vi "Calculate merit factor.vi"(8 "error in (no error)":errorcluster, 11 "DAQOrcaFlash in":refnum<class "DAQOrcaFlash.lvclass">) -> (0 "error out":errorcluster, 3 "DAQOrcaFlash out":refnum<class "DAQOrcaFlash.lvclass">)   [LabVIEW 2012, in "DAQOrcaFlash.lvclass"]
uses:
  DAQOrcaFlash.lvclass
  ROI options.ctl
  <vilib>/Distrio/Murmex/GenericMessage/GenericMessage.lvclass
  DAQOrcaFlash.lvclass/DAQOrcaFlash.ctl
  <vilib>/Analysis/6fits.llb/Curve Fitting Criteria.ctl
  <vilib>/Analysis/baseanly.llb/Mean (DBL).vi
  <vilib>/Analysis/NI_AALBase.lvlib
  <vilib>/vision/NI_Vision_Development_Module.lvlib
  <vilib>/Analysis/NI_AALPro.lvlib
  <vilib>/Distrio/Murmex/Message/Message.lvclass
  <vilib>/Distrio/Murmex/Murmex/Murmex.lvclass
panel:
  in  "amplitude guess":dbl=1.0
  in  "STD guess":dbl=0.1
  out "LP":T1(plugin-control)
  out "HP":dbl(graph)
  out "LP":dbl(graph)
  out "y2 2":dbl
  out "x2 2":dbl
  out "y1 2":dbl
  out "x1 2":dbl
  out "parameter guesses":dbl[](array[numeric])
  out "mean":dbl format="%0.2f"
  out "min value":dbl
  out "best fit parameters":dbl[](array[numeric])
  out "XY Graph":cluster{cdb[]}[](graph)
  out "size y":i32
  out "y2":dbl
  out "x2":dbl
  out "y1":dbl
  out "x1":dbl
  out "Runtime cluster.ROI Descriptor.Global Rectangle":i32[](array[numeric])
  out "offset":dbl
  out "standard deviation":dbl
  in  "ROI options 2":T2
  out "amplitude":dbl
  out "residue":dbl
  out "center":dbl
  out "Raw data":cluster{"Y":dbl[], "Y":dbl[]}[](graph)
  out "Gauss":cluster{"Y":dbl[], "Y":dbl[]}[](graph)
  out "HP":T1(plugin-control)
  out "MF":dbl(graph)
  # "y_min"
  # "y mean"
  # "ampl"
  # "STD"
  # "xo"
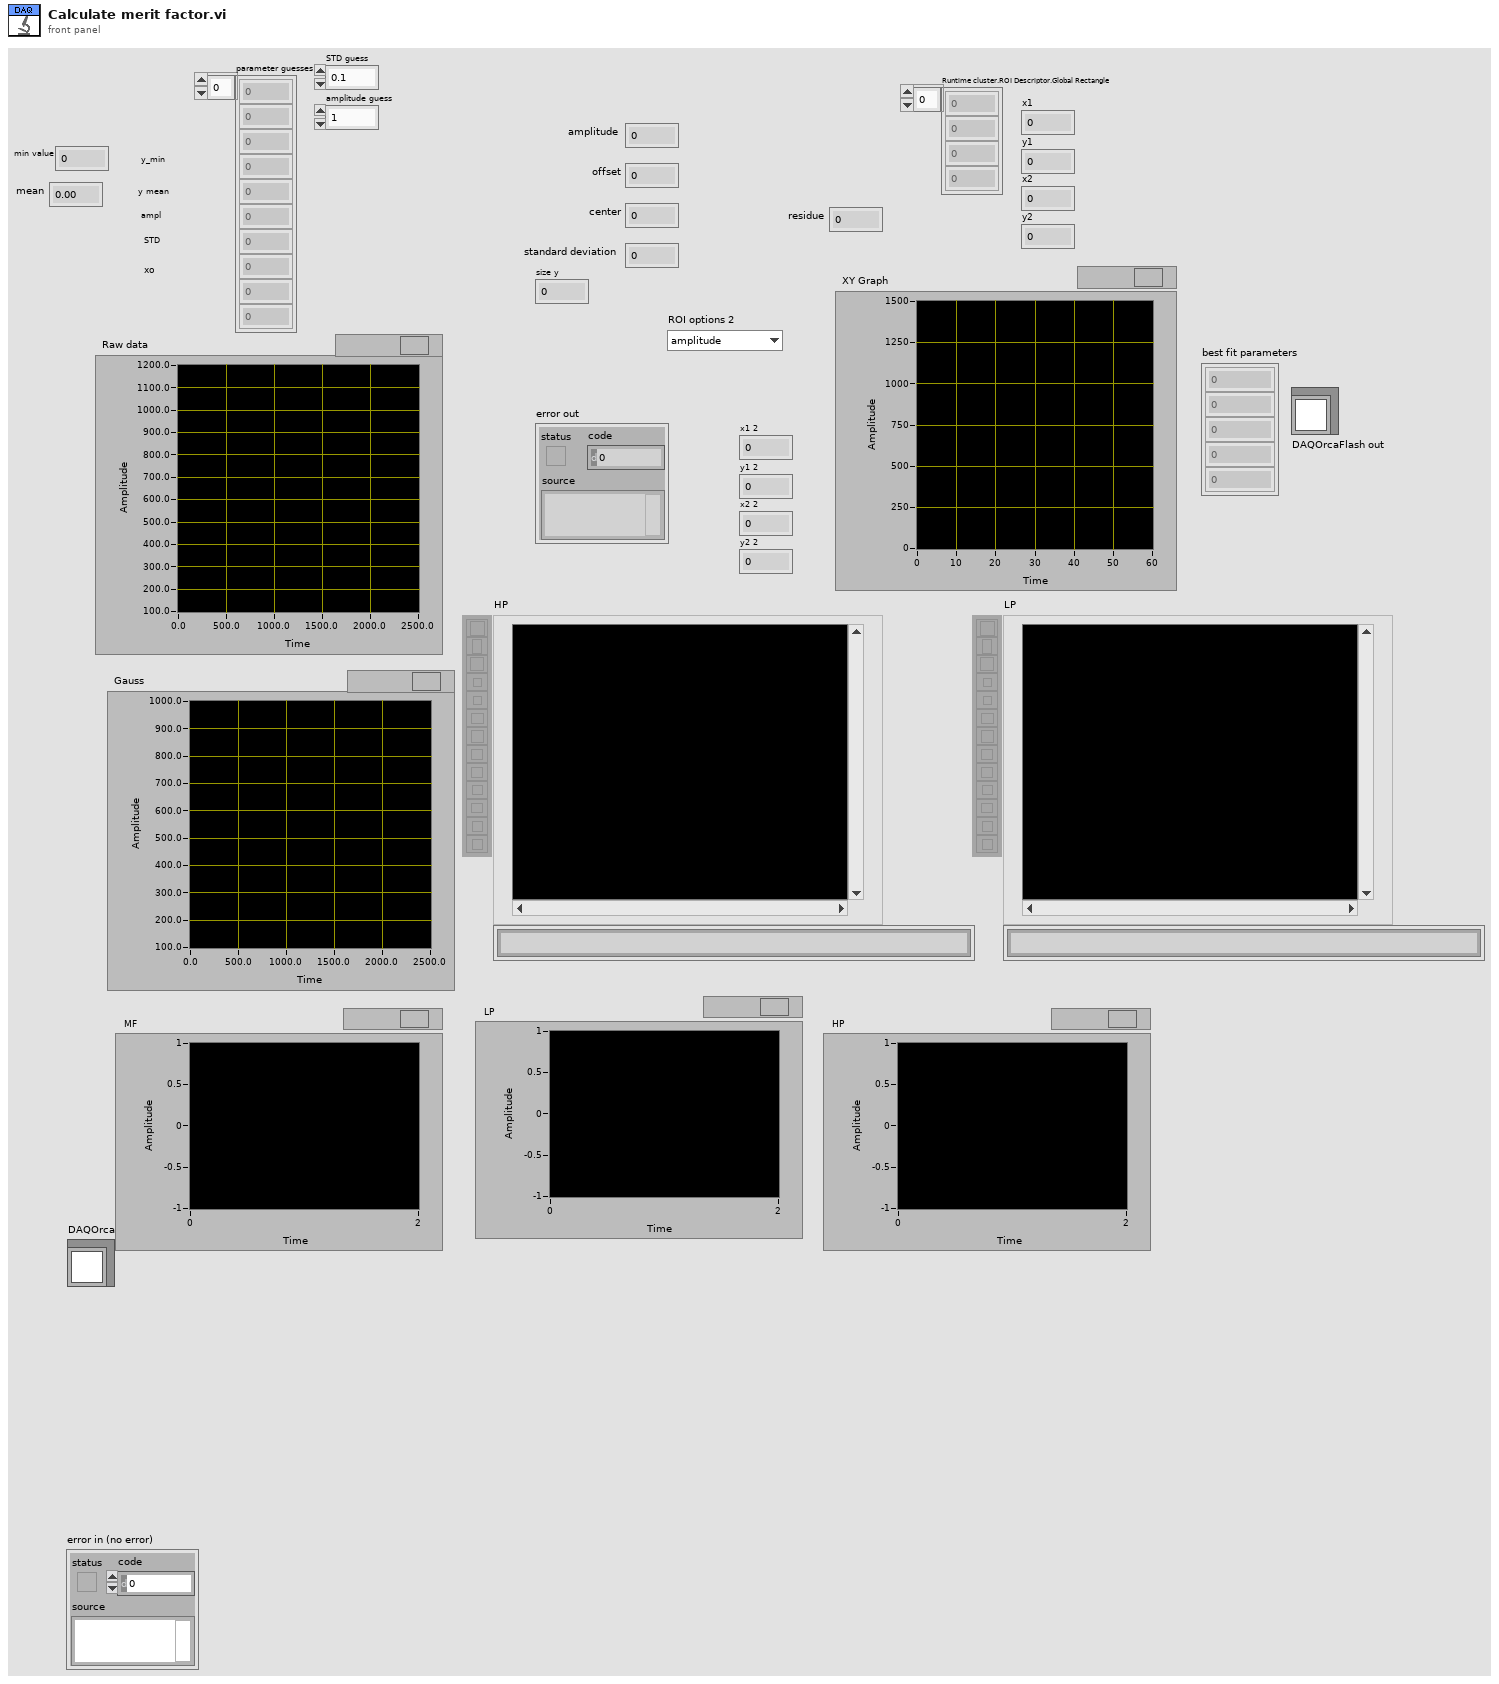
[diagram p1: front panel]
types:
  T1 = typedef "IMAQ Image.ctl" = refnum<image>
  T2 = typedef "DAQOrcaFlash.lvclass/ROI options.ctl" = enum16{"amplitude", "ERF", "residue", "amplitude/STD", "amplitude/offset"}
  T3 = cluster{"initial amplitude":dbl, "initial center":dbl, "initial standard deviation":dbl, "offset":dbl}
  T4 = cluster{"amp min":dbl, "amp max":dbl, "center min":dbl, "center max":dbl, "deviation min":dbl, "deviation max":dbl, "offset min":dbl, "offset max":dbl}
  T5 = typedef "Image Type" = u32
  T6 = typedef "DAQOrcaFlash.lvclass/merit_factor_type.ctl" = enum16{"full frame intensity", "ROI beads", "Weber contrast", "Michelson contrast", "RMS contrast", "Line profile analysis", "ROI analysis", "FFT", "SNR", "5% brightest"}
  T7 = typedef "ROI Descriptor" = cluster{"Global Rectangle":i32[], "Contours":cluster{"ID":enum32{"External", "Internal"}, "Type":u32, "Coordinates":i32[]}[]}
  T8 = cluster{"histogram":u32[], "Minimal Value":sgl, "Maximal Value":sgl, "Starting Value":sgl, "Interval Width":sgl, "Mean Value":sgl, "Standard  Variation":sgl, "Area (pixels)":i32}
  T9 = typedef "NI_AALPro.lvlib/Curve Fitting Criteria.ctl" = u16
  T10 = cluster{"Min":sgl, "Max":sgl, "Mean":sgl, "Std Dev":sgl, "Count":i32}
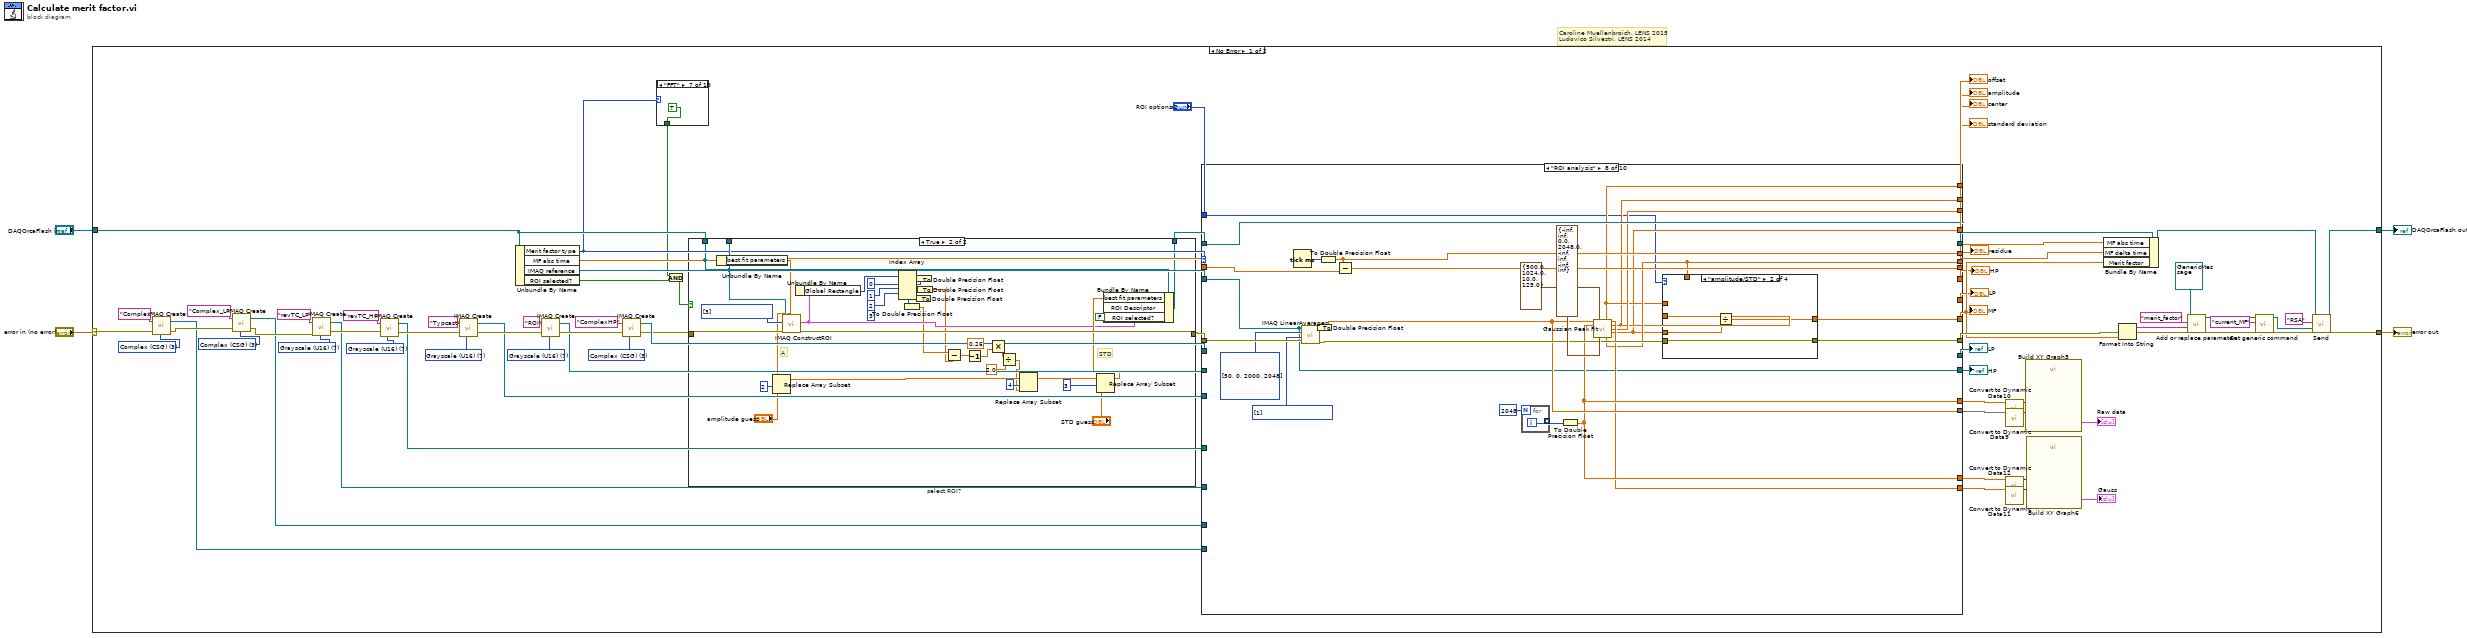
[diagram p0: block diagram]
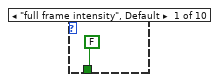
[diagram p2: hidden frame]
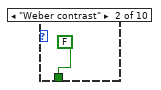
[diagram p3: hidden frame]
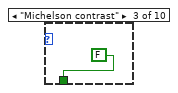
[diagram p4: hidden frame]
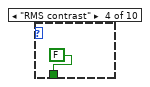
[diagram p5: hidden frame]
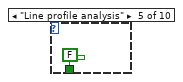
[diagram p6: hidden frame]
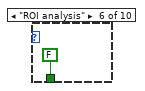
[diagram p7: hidden frame]
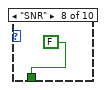
[diagram p8: hidden frame]
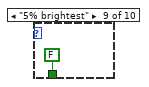
[diagram p9: hidden frame]
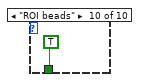
[diagram p10: hidden frame]
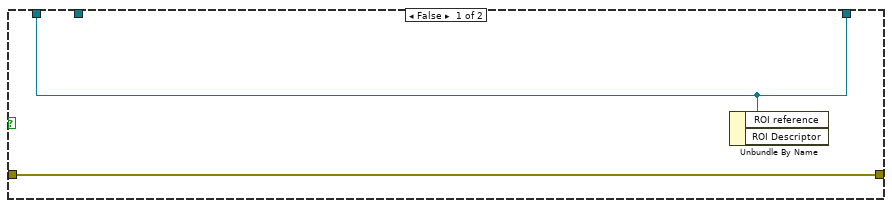
[diagram p11: hidden frame]
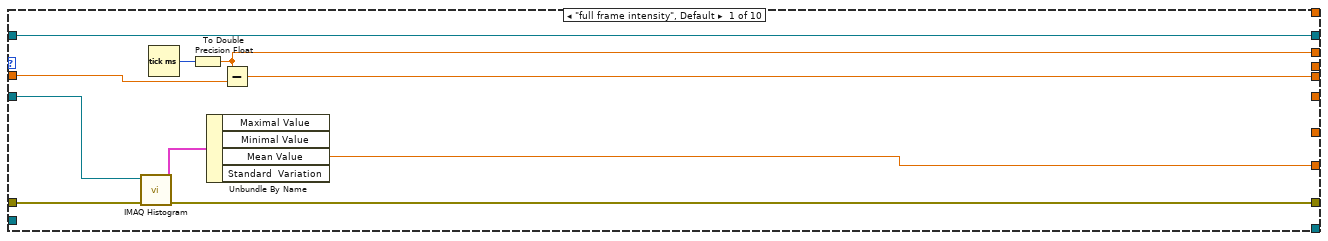
[diagram p12: hidden frame]
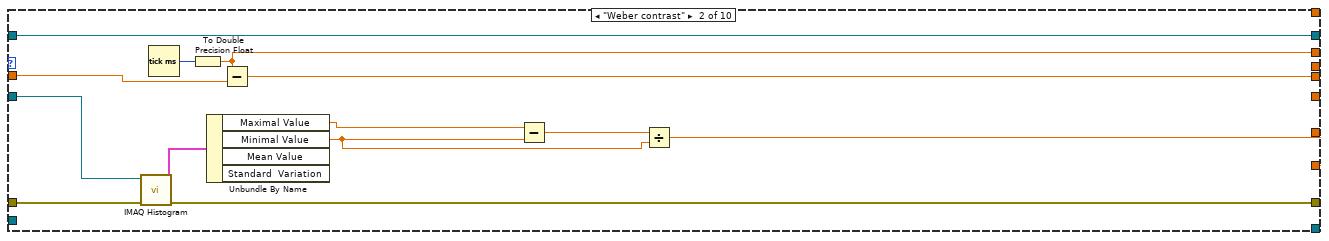
[diagram p13: hidden frame]
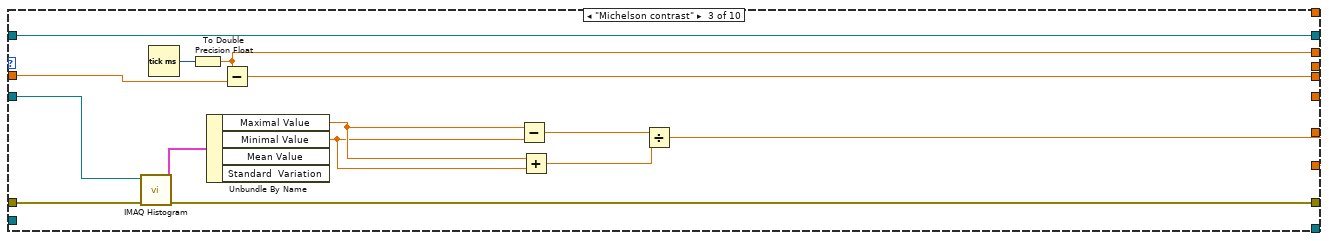
[diagram p14: hidden frame]
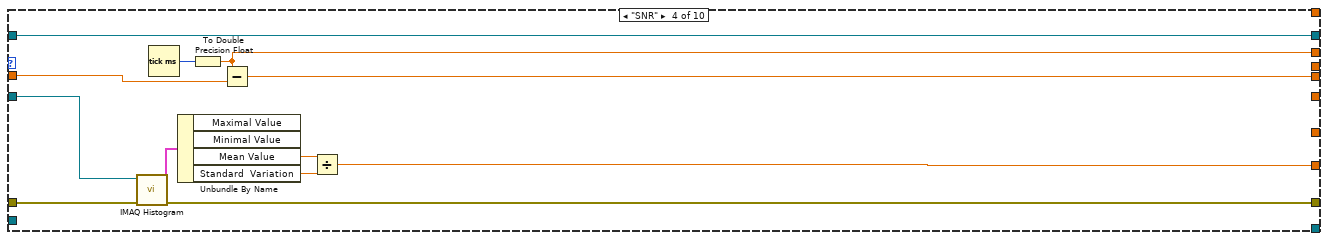
[diagram p15: hidden frame]
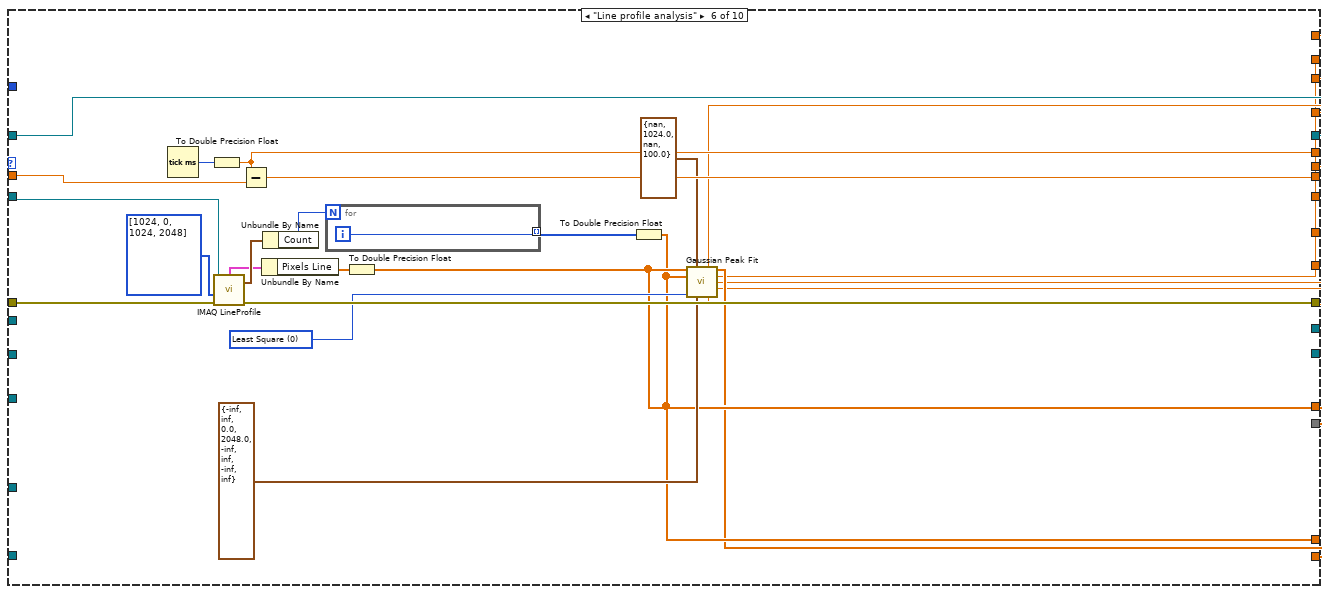
[diagram p17: hidden frame]
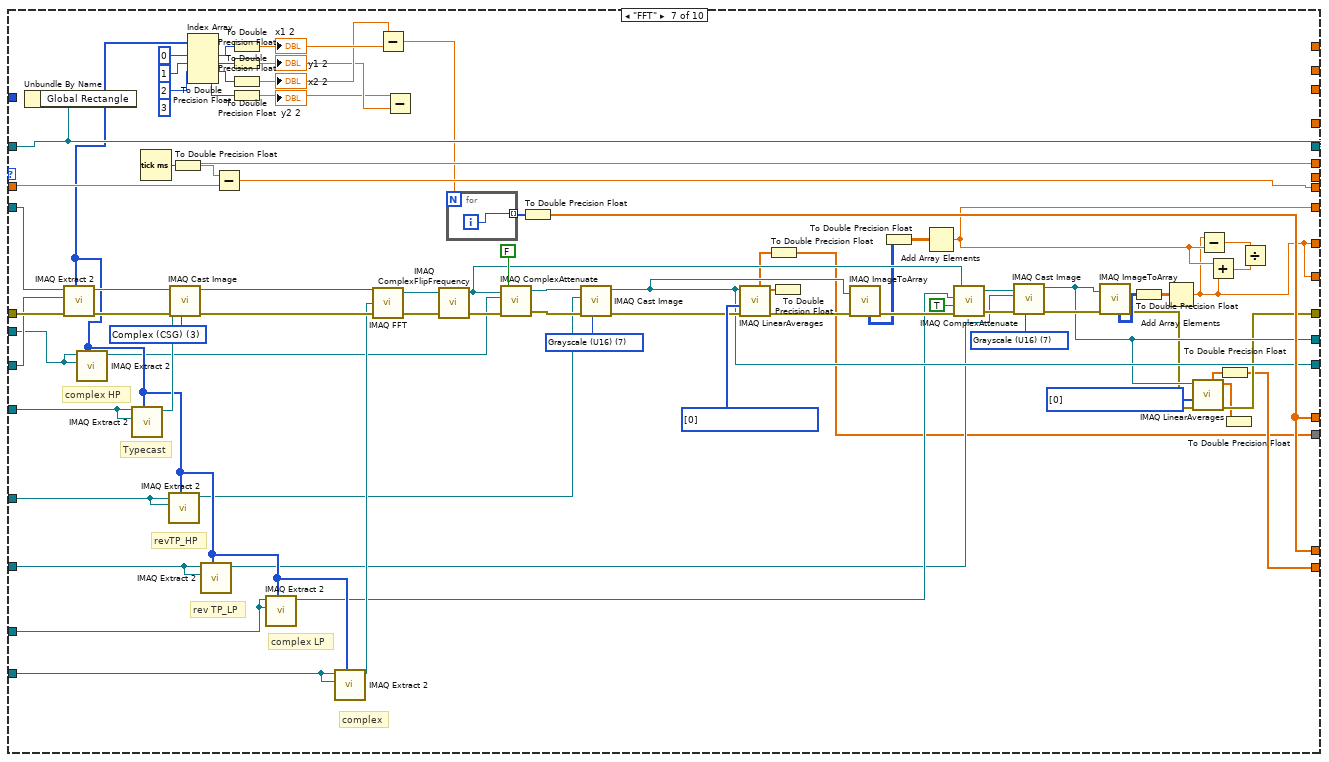
[diagram p18: hidden frame]
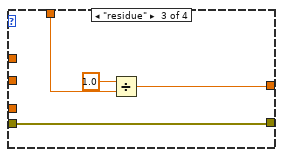
[diagram p20: hidden frame]
diagram:
  # "Caroline Muellenbroich, LENS 2015\nLudovico Silvestri, LENS 2014"
  n1 = case shown="No Error" "error in (no error)" {
    selector: "error in (no error)" -> [w11 w438]
    tunnel: [w67 w438] -> w4
    tunnel: "DAQOrcaFlash in" -> [w38 w439]
    tunnel: [w63 w439] -> w2
    frame No Error {
      w9 = T5 3 items=["Grayscale (U8)", "Grayscale (I16)", "Grayscale (SGL)", "Complex (CSG)", "RGB (U32)", "HSL (U32)", "RGB (U64)", "Grayscale (U16)"] ("Image Type")
      w14 = T5 3 items=["Grayscale (U8)", "Grayscale (I16)", "Grayscale (SGL)", "Complex (CSG)", "RGB (U32)", "HSL (U32)", "RGB (U64)", "Grayscale (U16)"] ("Image Type")
      w18 = T5 7 items=["Grayscale (U8)", "Grayscale (I16)", "Grayscale (SGL)", "Complex (CSG)", "RGB (U32)", "HSL (U32)", "RGB (U64)", "Grayscale (U16)"] ("Image Type")
      w22 = T5 7 items=["Grayscale (U8)", "Grayscale (I16)", "Grayscale (SGL)", "Complex (CSG)", "RGB (U32)", "HSL (U32)", "RGB (U64)", "Grayscale (U16)"] ("Image Type")
      w28 = T5 7 items=["Grayscale (U8)", "Grayscale (I16)", "Grayscale (SGL)", "Complex (CSG)", "RGB (U32)", "HSL (U32)", "RGB (U64)", "Grayscale (U16)"] ("Image Type")
      w31 = T5 7 items=["Grayscale (U8)", "Grayscale (I16)", "Grayscale (SGL)", "Complex (CSG)", "RGB (U32)", "HSL (U32)", "RGB (U64)", "Grayscale (U16)"] ("Image Type")
      w61 = T5 3 items=["Grayscale (U8)", "Grayscale (I16)", "Grayscale (SGL)", "Complex (CSG)", "RGB (U32)", "HSL (U32)", "RGB (U64)", "Grayscale (U16)"] ("Image Type")
      n2 = call "IMAQ Create"("Image Name"="Complex", "Image Type"=w9, "error in (no error)"=w11) -> ("New Image"=w8:T1, "error out"=w10:errorcluster)  [unwired: 2 in]
      n3 = call "IMAQ Create"("Image Name"="Complex_LP", "Image Type"=w14, "error in (no error)"=w10) -> ("New Image"=w13:T1, "error out"=w15:errorcluster)  [unwired: 2 in]
      n4 = call "IMAQ Create"("Image Name"="revTC_LP", "Image Type"=w18, "error in (no error)"=w15) -> ("New Image"=w17:T1, "error out"=w19:errorcluster)  [unwired: 2 in]
      n5 = call "IMAQ Create"("Image Name"="revTC_HP", "Image Type"=w22, "error in (no error)"=w19) -> ("New Image"=w21:T1, "error out"=w23:errorcluster)  [unwired: 2 in]
      n6 = call "IMAQ Create"("Image Name"="Typcast", "Image Type"=w28, "error in (no error)"=w23) -> ("New Image"=w25:T1, "error out"=w26:errorcluster)  [unwired: 2 in]
      n7 = Unbundle By Name(w38) -> ("Merit factor type"=w36:T6, "MF abs time"=w80:dbl, "IMAQ reference"=w55:T1, "ROI selected?"=w35:bool)
      n8 = call "IMAQ Create"("Image Name"="ROI", "Image Type"=w31, "error in (no error)"=w26) -> ("New Image"=w29:T1, "error out"=w30:errorcluster)  [unwired: 2 in]
      n9 = call "IMAQ Create"("Image Name"="ComplexHP", "Image Type"=w61, "error in (no error)"=w30) -> ("New Image"=w60:T1, "error out"=w57:errorcluster)  [unwired: 2 in]
      n10 = case shown="\"FFT\"" w36 {
        tunnel: [FALSE FALSE FALSE FALSE FALSE FALSE TRUE FALSE FALSE TRUE] -> w34
        frame "full frame intensity", Default {
        }
        frame "Weber contrast" {
        }
        frame "Michelson contrast" {
        }
        frame "RMS contrast" {
        }
        frame "Line profile analysis" {
        }
        frame "ROI analysis" {
        }
        frame "FFT" {
        }
        frame "SNR" {
        }
        frame "5% brightest" {
        }
        frame "ROI beads" {
        }
      }
      n11 = And(x=w34, y=w35) -> (x .and. y?=w33:bool)
      n12 = case "select ROI?" shown="True" w33 {
        tunnel: w57 -> [w92 w124]
        tunnel: [w92 w123] -> w56
        tunnel: w55 -> [_ w122]
        tunnel: w38 -> [w91 w119]
        tunnel: [w91 w121] -> w37
        frame False {
          n13 = Unbundle By Name(w91) -> ()  [unwired: 2 out]
        }
        frame True {
          (unwired) 3 ("index")
          w125 = u32[] [3] items=["No Selection", "Point", "Line", "Rectangle", "Oval", "Polygon", "Freehand Region", "Annulus", "Zoom", "Pan", "Broken Line", "Freehand Line", "Rotated Rectangle"] ("Tools")
          # "A"
          # "STD"
          n14 = Unbundle By Name(w119) -> ("best fit parameters"=w114:dbl[])
          n15 = Replace Array Subset(array=w114, new element="amplitude guess", index=2) -> (w99:dbl[])
          n16 = call "IMAQ ConstructROI"("error in (no error)"=w124, "Tools"=w125, "Image"=w122) -> ("error out"=w123:errorcluster, "ROI Descriptor Out"=w112:T7)  [unwired: 5 in, 2 out]
          n17 = Unbundle By Name(w112) -> ("Global Rectangle"=w104:i32[])
          n18 = Index Array(array=w104, index #1=0 ("index"), index #2=1 ("index"), index #3=2 ("index")) -> (element #1=w111:i32, element #2=w110:i32, element #3=w108:i32, element #4=w109:i32)  [unwired: 1 in]
          n19 = To Double Precision Float(number=w109) -> (double precision float=w103:dbl)
          n20 = To Double Precision Float(number=w108) -> ()  [unwired: 1 out]
          n21 = To Double Precision Float(number=w111) -> ()  [unwired: 1 out]
          n22 = To Double Precision Float(number=w110) -> (double precision float=w102:dbl)
          n23 = Subtract(x=w103, y=w102) -> (x-y=w101:dbl)
          n24 = Decrement(x=w101) -> (x-1=w94:dbl)
          n25 = Multiply(x=0.26, y=w94) -> (x*y=w93:dbl)
          n26 = Divide(x=w93, y=2.0) -> (x/y=w96:dbl)
          n27 = Replace Array Subset(array=w99, new element=w96, index=4) -> (w98:dbl[])
          n28 = Replace Array Subset(array=w98, new element="STD guess", index=3) -> (w113:dbl[])
          n29 = Bundle By Name(cluster=w119, "best fit parameters"=w113, "ROI Descriptor"=w112, "ROI selected?"=FALSE ("Runtime cluster.ROI selected?")) -> (w121:refnum<class "DAQOrcaFlash.lvclass">)
        }
      }
      n30 = case shown="\"ROI analysis\"" w36 {
        tunnel: [w129 w142 w156 w168 w175 w199 w229 w292 w363 w418] -> w74
        tunnel: w56 -> [w130 w143 w157 w169 w175 w201 w264 w299 w355 w417]
        tunnel: w37 -> [w132 w145 w159 w171 w176 w194 w265 w305 w325 w416]
        tunnel: [w132 w145 w159 w171 w176 w194 w265 w305 w324 w416] -> w78
        tunnel: w80 -> [w135 w148 w162 w174 _ w190 w266 w302 w370 w415]
        tunnel: [w134 w147 w161 w173 _ w189 w259 w301 w369 w414] -> w79
        tunnel: [w126 w136 w152 w163 _ w177 w203 w291 w362 w413] -> w62
        tunnel: [w131 w144 w158 w170 _ w188 w257 w300 w368 w412] -> w77
        tunnel: w55 -> [w128 w141 w155 w167 _ w200 w262 w281 w346 _]
        tunnel: w60 -> [_ _ _ _ _ _ w224 _ _ _]
        tunnel: [_ _ _ _ _ _ w239 w281 w345 _] -> w58
        tunnel: [_ _ _ _ _ w182 w253 w289 w321 _] -> w48
        tunnel: [_ _ _ _ _ w183 w206 w290 w327 _] -> w47
        tunnel: [_ _ _ _ _ w182 w253 w289 w321 _] -> w46
        tunnel: [_ _ _ _ _ w181 w207 w288 w329 _] -> w45
        tunnel: [_ _ _ _ _ w184 _ w285 w361 _] -> w44
        tunnel: [_ _ _ _ _ w177 _ w284 w360 _] -> w43
        tunnel: [_ _ _ _ _ w180 _ w286 w359 _] -> w42
        tunnel: [_ _ _ _ _ w179 _ w283 w358 _] -> w41
        tunnel: [_ _ _ _ _ w178 _ w287 w357 _] -> w40
        tunnel: "ROI options 2" -> [_ _ _ _ _ _ _ w282 w356 _]
        tunnel: w29 -> [_ _ _ _ _ _ w263 _ w343 _]
        tunnel: w25 -> [_ _ _ _ _ _ w223 _ _ _]
        tunnel: w21 -> [_ _ _ _ _ _ w221 _ _ _]
        tunnel: w17 -> [_ _ _ _ _ _ w220 _ _ _]
        tunnel: w13 -> [_ _ _ _ _ _ w219 _ _ _]
        tunnel: w8 -> [_ _ _ _ _ _ w218 _ _ _]
        tunnel: [_ _ _ _ _ _ w231 _ _ _] -> w7
        tunnel: [_ _ _ _ _ _ w204 _ _ _] -> w6
        tunnel: [_ _ _ _ _ _ w203 _ _ _] -> w5
        frame "full frame intensity", Default {
          n31 = call "IMAQ Histogram"("error in (no error)"=w130, "Image"=w128) -> ("error out"=w129:errorcluster, "Histogram Report"=w127:T8)  [unwired: 8 in]
          n32 = Tick Count (ms)() -> (millisecond timer value=w133:u32)
          n33 = To Double Precision Float(number=w133) -> (double precision float=w131:dbl)
          n34 = Unbundle By Name(w127) -> ("Mean Value"=w126:sgl)  [unwired: 3 out]
          n35 = Subtract(x=w131, y=w135) -> (x-y=w134:dbl)
        }
        frame "Weber contrast" {
          n36 = call "IMAQ Histogram"("error in (no error)"=w143, "Image"=w141) -> ("error out"=w142:errorcluster, "Histogram Report"=w140:T8)  [unwired: 8 in]
          n37 = Tick Count (ms)() -> (millisecond timer value=w146:u32)
          n38 = To Double Precision Float(number=w146) -> (double precision float=w144:dbl)
          n39 = Unbundle By Name(w140) -> ("Maximal Value"=w139:sgl, "Minimal Value"=w137:sgl)  [unwired: 2 out]
          n40 = Subtract(x=w144, y=w148) -> (x-y=w147:dbl)
          n41 = Subtract(x=w139, y=w137) -> (x-y=w138:sgl)
          n42 = Divide(x=w138, y=w137) -> (x/y=w136:sgl)
        }
        frame "Michelson contrast" {
          n43 = call "IMAQ Histogram"("error in (no error)"=w157, "Image"=w155) -> ("error out"=w156:errorcluster, "Histogram Report"=w154:T8)  [unwired: 8 in]
          n44 = Tick Count (ms)() -> (millisecond timer value=w160:u32)
          n45 = To Double Precision Float(number=w160) -> (double precision float=w158:dbl)
          n46 = Unbundle By Name(w154) -> ("Maximal Value"=w151:sgl, "Minimal Value"=w150:sgl)  [unwired: 2 out]
          n47 = Subtract(x=w158, y=w162) -> (x-y=w161:dbl)
          n48 = Subtract(x=w151, y=w150) -> (x-y=w153:sgl)
          n49 = Add(x=w151, y=w150) -> (x+y=w149:sgl)
          n50 = Divide(x=w153, y=w149) -> (x/y=w152:sgl)
        }
        frame "SNR" {
          n51 = call "IMAQ Histogram"("error in (no error)"=w169, "Image"=w167) -> ("error out"=w168:errorcluster, "Histogram Report"=w166:T8)  [unwired: 8 in]
          n52 = Tick Count (ms)() -> (millisecond timer value=w172:u32)
          n53 = Unbundle By Name(w166) -> ("Mean Value"=w165:sgl, "Standard  Variation"=w164:sgl)  [unwired: 2 out]
          n54 = To Double Precision Float(number=w172) -> (double precision float=w170:dbl)
          n55 = Subtract(x=w170, y=w174) -> (x-y=w173:dbl)
          n56 = Divide(x=w165, y=w164) -> (x/y=w163:sgl)
        }
        frame "RMS contrast" {
        }
        frame "Line profile analysis" {
          w187 = T9 0 items=["Least Square", "Least Absolute Residual", "Bisquare"] ("method")
          n57 = Tick Count (ms)() -> (millisecond timer value=w191:u32)
          n58 = To Double Precision Float(number=w191) -> (double precision float=w188:dbl)
          n59 = call "IMAQ LineProfile"("error in (no error)"=w201, "Line Coordinates"=i32[] [1024, 0, 1024, 2048], "Image"=w200) -> ("error out"=w199:errorcluster, "Line Graph"=w196:cluster{"x0":sgl, "dx":sgl, "Pixels Line":sgl[]}, "Line Information"=w198:T10)  [unwired: 2 in, 1 out]
          n60 = Subtract(x=w188, y=w190) -> (x-y=w189:dbl)
          n61 = Unbundle By Name(w196) -> ("Pixels Line"=w195:sgl[])
          n62 = Unbundle By Name(w198) -> ("Count"=w193:i32)
          n63 = for {
            N: w193 -> [_]
            tunnel: [w202] -> w192 mode=indexing
            i -> [w202]
          }
          n64 = To Double Precision Float(number=w195) -> (double precision float=w183:dbl[])
          n65 = To Double Precision Float(number=w192) -> (double precision float=w182:dbl[])
          n66 = call <vilib>:"Gaussian Peak Fit.vi"("Y"=w183, "initial guess"=T3 {"initial amplitude"=nan, "initial center"=1024.0, "initial standard deviation"=nan, "offset"=100.0}, "X"=w182, "method"=w187, "parameter bounds"=T4 {"amp min"=-inf, "amp max"=inf, "center min"=0.0, "center max"=2048.0, "deviation min"=-inf, "deviation max"=inf, "offset min"=-inf, "offset max"=inf}) -> ("offset"=w184:dbl, "Best Gaussian Fit"=w181:dbl[], "amplitude"=w177:dbl, "center"=w180:dbl, "standard deviation"=w179:dbl, "residue"=w178:dbl)  [unwired: 4 in, 1 out]
        }
        frame "FFT" {
          w228 = i32[] [0] items=["X Axis Averages", "Y Axis Averages", "X + Y Axis Averages", "X - Y Axis Averages"] ("Averages")
          w243 = T5 7 items=["Grayscale (U8)", "Grayscale (I16)", "Grayscale (SGL)", "Complex (CSG)", "RGB (U32)", "HSL (U32)", "RGB (U64)", "Grayscale (U16)"] ("Image Type")
          w254 = T5 7 items=["Grayscale (U8)", "Grayscale (I16)", "Grayscale (SGL)", "Complex (CSG)", "RGB (U32)", "HSL (U32)", "RGB (U64)", "Grayscale (U16)"] ("Image Type")
          w261 = i32[] [0] items=["X Axis Averages", "Y Axis Averages", "X + Y Axis Averages", "X - Y Axis Averages"] ("Averages")
          (unwired) 3 ("index")
          w278 = T5 3 items=["Grayscale (U8)", "Grayscale (I16)", "Grayscale (SGL)", "Complex (CSG)", "RGB (U32)", "HSL (U32)", "RGB (U64)", "Grayscale (U16)"] ("Image Type")
          # "complex"
          # "complex LP"
          # "rev TP_LP"
          # "revTP_HP"
          # "Typecast"
          # "complex HP"
          n67 = Unbundle By Name(w265) -> ("Global Rectangle"=w217:i32[])
          n68 = call "IMAQ Extract 2"("Optional Rectangle"=w217, "error in (no error)"=w264, "Image Dst"=w263, "Image Src"=w262) -> ("error out"=w226:errorcluster, "Image Dst Out"=w227:T1)  [unwired: 6 in]
          n69 = call "IMAQ Extract 2"("Optional Rectangle"=w217, "Image Dst"=w224, "Image Src"=w224) -> ("Image Dst Out"=w214:T1)  [unwired: 7 in, 1 out]
          n70 = call "IMAQ Extract 2"("Optional Rectangle"=w217, "Image Dst"=w223, "Image Src"=w223) -> ("Image Dst Out"=w222:T1)  [unwired: 7 in, 1 out]
          n71 = Tick Count (ms)() -> (millisecond timer value=w258:u32)
          n72 = call "IMAQ Extract 2"("Optional Rectangle"=w217, "Image Dst"=w221, "Image Src"=w221) -> ("Image Dst Out"=w213:T1)  [unwired: 7 in, 1 out]
          n73 = call "IMAQ Cast Image"("Image Type"=w278, "error in (no error)"=w226, "Image Dst"=w222, "Image Src"=w227) -> ("error out"=w225:errorcluster, "Image Dst Out"=w216:T1)  [unwired: 6 in]
          n74 = To Double Precision Float(number=w258) -> (double precision float=w257:dbl)
          n75 = Index Array(array=w217, index #1=0 ("index"), index #2=1 ("index"), index #3=2 ("index")) -> (element #1=w270:i32, element #2=w271:i32, element #3=w273:i32, element #4=w272:i32)  [unwired: 1 in]
          n76 = call "IMAQ Extract 2"("Optional Rectangle"=w217, "Image Dst"=w220, "Image Src"=w220) -> ("Image Dst Out"=w211:T1)  [unwired: 7 in, 1 out]
          n77 = Subtract(x=w257, y=w266) -> (x-y=w259:dbl)
          n78 = To Double Precision Float(number=w270) -> (double precision float=w269:dbl)
          "x1 2" <- w269
          n79 = To Double Precision Float(number=w271) -> (double precision float=w267:dbl)
          "y1 2" <- w267
          n80 = To Double Precision Float(number=w273) -> (double precision float=w268:dbl)
          "x2 2" <- w268
          n81 = To Double Precision Float(number=w272) -> (double precision float=w256:dbl)
          "y2 2" <- w256
          n82 = call "IMAQ Extract 2"("Optional Rectangle"=w217, "Image Dst"=w219, "Image Src"=w219) -> ("Image Dst Out"=w212:T1)  [unwired: 7 in, 1 out]
          n83 = call "IMAQ Extract 2"("Optional Rectangle"=w217, "Image Dst"=w218, "Image Src"=w218) -> ("Image Dst Out"=w215:T1)  [unwired: 7 in, 1 out]
          n84 = call "IMAQ FFT"("error in (no error)"=w225, "Image Dst"=w215, "Image Src"=w216) -> ("error out"=w252:errorcluster, "Image Dst Out"=w251:T1)  [unwired: 1 in]
          n85 = Subtract(x=w268, y=w269) -> (x-y=w205:dbl)
          n86 = Subtract(x=w256, y=w267) -> ()  [unwired: 1 out]
          n87 = call "IMAQ ComplexFlipFrequency"("error in (no error)"=w252, "Image Src"=w251) -> ("error out"=w250:errorcluster, "Image Dst Out"=w246:T1)  [unwired: 2 in]
          n88 = for {
            N: w205 -> [_]
            tunnel: [w279] -> w277 mode=indexing
            i -> [w279]
          }
          n89 = call "IMAQ ComplexAttenuate"("error in (no error)"=w250, "Low pass/High pass (Low pass)"=FALSE, "Image Dst"=w214, "Image Src"=w246) -> ("error out"=w249:errorcluster, "Image Dst Out"=w248:T1)  [unwired: 1 in]
          n90 = To Double Precision Float(number=w277) -> (double precision float=w253:dbl[])
          n91 = call "IMAQ Cast Image"("Image Type"=w254, "error in (no error)"=w249, "Image Dst"=w213, "Image Src"=w248) -> ("error out"=w255:errorcluster, "Image Dst Out"=w239:T1)  [unwired: 6 in]
          n92 = call "IMAQ LinearAverages"("error in (no error)"=w255, "Averages"=w261, "Image Src"=w239) -> ("error out"=w241:errorcluster, "Y Axis Averages"=w260:sgl[], "X Axis Averages"=w210:sgl[])  [unwired: 4 in, 2 out]
          n93 = To Double Precision Float(number=w210) -> (double precision float=w206:dbl[])
          n94 = To Double Precision Float(number=w260) -> ()  [unwired: 1 out]
          n95 = call "IMAQ ImageToArray"("error in (no error)"=w241, "Image"=w239) -> ("Image Pixels (U16)"=w235:u16[][], "error out"=w240:errorcluster)  [unwired: 2 in, 3 out]
          n96 = To Double Precision Float(number=w235) -> (double precision float=w238:dbl[][])
          n97 = Add Array Elements(numeric array=w238) -> (sum=w204:dbl)
          n98 = call "IMAQ ComplexAttenuate"("error in (no error)"=w240, "Low pass/High pass (Low pass)"=TRUE, "Image Dst"=w212, "Image Src"=w246) -> ("error out"=w245:errorcluster, "Image Dst Out"=w244:T1)  [unwired: 1 in]
          n99 = call "IMAQ Cast Image"("Image Type"=w243, "error in (no error)"=w245, "Image Dst"=w211, "Image Src"=w244) -> ("error out"=w237:errorcluster, "Image Dst Out"=w231:T1)  [unwired: 6 in]
          n100 = call "IMAQ ImageToArray"("error in (no error)"=w237, "Image"=w231) -> ("Image Pixels (U16)"=w234:u16[][], "error out"=w230:errorcluster)  [unwired: 2 in, 3 out]
          n101 = To Double Precision Float(number=w234) -> (double precision float=w236:dbl[][])
          n102 = Add Array Elements(numeric array=w236) -> (sum=w203:dbl)
          n103 = call "IMAQ LinearAverages"("error in (no error)"=w230, "Averages"=w228, "Image Src"=w231) -> ("error out"=w229:errorcluster, "Y Axis Averages"=w209:sgl[], "X Axis Averages"=w208:sgl[])  [unwired: 4 in, 2 out]
          n104 = Subtract(x=w203, y=w204) -> (x-y=w232:dbl)
          n105 = Add(x=w204, y=w203) -> (x+y=w233:dbl)
          n106 = To Double Precision Float(number=w208) -> (double precision float=w207:dbl[])
          n107 = To Double Precision Float(number=w209) -> ()  [unwired: 1 out]
          n108 = Divide(x=w232, y=w233) -> ()  [unwired: 1 out]
        }
        frame "ROI analysis" {
          w297 = i32[] [1] items=["X Axis Averages", "Y Axis Averages", "X + Y Axis Averages", "X - Y Axis Averages"] ("Averages")
          n109 = Tick Count (ms)() -> (millisecond timer value=w303:u32)
          n110 = call "IMAQ LinearAverages"("error in (no error)"=w299, "Averages"=w297, "Optional Rectangle"=i32[] [50, 0, 2000, 2048], "Image Src"=w281) -> ("error out"=w293:errorcluster, "Y Axis Averages"=w295:sgl[])  [unwired: 3 in, 3 out]
          n111 = To Double Precision Float(number=w295) -> (double precision float=w290:dbl[])
          n112 = To Double Precision Float(number=w303) -> (double precision float=w300:dbl)
          n113 = Subtract(x=w300, y=w302) -> (x-y=w301:dbl)
          n114 = for {
            N: 2048 -> [_]
            tunnel: [w320] -> w304 mode=indexing
            i -> [w320]
          }
          n115 = To Double Precision Float(number=w304) -> (double precision float=w289:dbl[])
          n116 = call <vilib>:"Gaussian Peak Fit.vi"("Y"=w290, "initial guess"=T3 {"initial amplitude"=500.0, "initial center"=1024.0, "initial standard deviation"=10.0, "offset"=125.0}, "X"=w289, "parameter bounds"=T4 {"amp min"=-inf, "amp max"=inf, "center min"=0.0, "center max"=2048.0, "deviation min"=-inf, "deviation max"=inf, "offset min"=-inf, "offset max"=inf}) -> ("offset"=w285:dbl, "Best Gaussian Fit"=w288:dbl[], "amplitude"=w284:dbl, "center"=w286:dbl, "standard deviation"=w283:dbl, "residue"=w287:dbl)  [unwired: 5 in, 1 out]
          n117 = case shown="\"amplitude/STD\"" w282 {
            tunnel: w293 -> [w306 w311 w313 w316]
            tunnel: [w306 w311 w313 w316] -> w292
            tunnel: [w307 w308 w314 w317] -> w291
            tunnel: w284 -> [w307 w310 _ w319]
            tunnel: w283 -> [_ w309 _ _]
            tunnel: w285 -> [_ _ _ w318]
            tunnel: w287 -> [_ _ w315 _]
            frame "amplitude", Default {
            }
            frame "amplitude/STD" {
              n118 = Divide(x=w310, y=w309) -> (x/y=w308:dbl)
            }
            frame "residue" {
              n119 = Divide(x=1.0, y=w315) -> (x/y=w314:dbl)
            }
            frame "amplitude/offset" {
              n120 = Divide(x=w319, y=w318) -> (x/y=w317:dbl)
            }
          }
        }
        frame "ROI beads" {
          w367 = i32[] [1] items=["X Axis Averages", "Y Axis Averages", "X + Y Axis Averages", "X - Y Axis Averages"] ("Averages")
          n121 = Unbundle By Name(w325) -> ("best fit parameters"=w326:dbl[], "Global Rectangle"=w332:i32[])
          "Runtime cluster.ROI Descriptor.Global Rectangle" <- w332
          n122 = Tick Count (ms)() -> (millisecond timer value=w371:u32)
          n123 = To Double Precision Float(number=w371) -> (double precision float=w368:dbl)
          n124 = Index Array(array=w332, index #1=0 ("index"), index #2=1 ("index"), index #3=2 ("index"), index #4=3 ("index")) -> (element #1=w342:i32, element #2=w347:i32, element #3=w349:i32, element #4=w348:i32)
          n125 = Subtract(x=w368, y=w370) -> (x-y=w369:dbl)
          n126 = To Double Precision Float(number=w348) -> (double precision float=w340:dbl)
          "y2" <- w340
          n127 = To Double Precision Float(number=w349) -> (double precision float=w339:dbl)
          "x2" <- w339
          n128 = To Double Precision Float(number=w342) -> (double precision float=w341:dbl)
          "x1" <- w341
          n129 = To Double Precision Float(number=w347) -> (double precision float=w333:dbl)
          "y1" <- w333
          n130 = Subtract(x=w339, y=w341) -> ()  [unwired: 1 out]
          n131 = Subtract(x=w340, y=w333) -> (x-y=w328:dbl)
          n132 = call "IMAQ Extract 2"("Optional Rectangle"=w332, "error in (no error)"=w355, "Image Dst"=w343, "Image Src"=w346) -> ("error out"=w354:errorcluster, "Image Dst Out"=w345:T1)  [unwired: 6 in]
          n133 = call "IMAQ LinearAverages"("error in (no error)"=w354, "Averages"=w367, "Image Src"=w345) -> ("error out"=w364:errorcluster, "Y Axis Averages"=w366:sgl[], "X Axis Averages"=w331:sgl[])  [unwired: 4 in, 2 out]
          n134 = for {
            N: w328 -> [_]
            tunnel: [w410] -> w321 mode=indexing
            i -> [w409]
            n135 = To Double Precision Float(number=w409) -> (double precision float=w408:dbl)
            n136 = Multiply(x=0.26, y=w408) -> (x*y=w410:dbl)
          }
          n137 = To Double Precision Float(number=w331) -> ()  [unwired: 1 out]
          n138 = To Double Precision Float(number=w366) -> (double precision float=w330:dbl[])
          n139 = Reverse 1D Array(array=w330) -> (reversed array=w327:dbl[])
          n140 = Array Size(array=w327) -> (size(s)=→"size y":i32)
          n141 = Array Max & Min(array=w327) -> (min value=w337:dbl)  [unwired: 3 out]
          "min value" <- w337
          n142 = call-poly <vilib>:"Mean.vi"("X"=w327) -> ("mean"=w334:dbl)  [unwired: 1 out]
          "mean" <- w334
          n143 = call <vilib>:"Gaussian Peak Fit.vi"("Y"=w327, "X"=w321, "parameter bounds"=T4 {"amp min"=-inf, "amp max"=inf, "center min"=0.0, "center max"=inf, "deviation min"=-inf, "deviation max"=inf, "offset min"=-inf, "offset max"=inf}) -> ("offset"=w361:dbl, "Best Gaussian Fit"=w329:dbl[], "amplitude"=w360:dbl, "center"=w359:dbl, "standard deviation"=w358:dbl, "residue"=w357:dbl)  [unwired: 6 in, 1 out]
          n144 = Replace Array Subset(array=w326, new element=w337, index=0) -> (w336:dbl[])
          n145 = Replace Array Subset(array=w336, new element=w334, index=1) -> (w322:dbl[])
          "parameter guesses" <- w322
          n146 = case shown="\"ERF\"" w356 {
            tunnel: w364 -> [w372 w377 w379 w383 w404]
            tunnel: [w372 w377 w379 w388 w404] -> w363
            tunnel: [w373 w374 w380 w384 w405] -> w362
            tunnel: w360 -> [w373 w376 _ _ w407]
            tunnel: w358 -> [_ w375 _ _ _]
            tunnel: w361 -> [_ _ _ _ w406]
            tunnel: w357 -> [_ _ w381 _ _]
            tunnel: w321 -> [_ _ _ w387 _]
            tunnel: w327 -> [_ _ _ w386 _]
            tunnel: w322 -> [_ _ _ w385 _]
            tunnel: [_ _ _ w382 _] -> w323
            frame "amplitude", Default {
            }
            frame "amplitude/STD" {
              n147 = Divide(x=w376, y=w375) -> (x/y=w374:dbl)
            }
            frame "residue" {
              n148 = Divide(x=1.0, y=w381) -> (x/y=w380:dbl)
            }
            frame "ERF" {
              n149 = case shown="No Error" w383 {
                selector: w383 -> [w393 w403]
                tunnel: [w389 w403] -> w388
                tunnel: w387 -> [w398 _]
                tunnel: w386 -> [w397 _]
                tunnel: [w396 _] -> w382
                tunnel: w385 -> [w394 _]
                tunnel: [w391 _] -> w384
                frame No Error {
                  n150 = call "Linespread_Function.vi"("error in (no error)"=w393, "Paramter guess"=w394, "y"=w397, "x"=w398) -> ("error out"=w392:errorcluster, "XY Graph"=→"XY Graph":cluster{cdb[]}[], "best fit parameters"=w396:dbl[])  [unwired: 5 in]
                  n151 = Index Array(array=w396, index=3) -> (element=w390:dbl)
                  n152 = case shown="No Error" w392 {
                    selector: w392 -> [w400 _]
                    tunnel: [w401 _] -> w391
                    tunnel: w390 -> [w401 _]
                    tunnel: [w400 errorcluster {"status"=FALSE, "code"=0, "source"=""} ("error constant")] -> w389
                    frame No Error {
                    }
                    frame Error {
                    }
                  }
                }
                frame Error {
                }
              }
              "best fit parameters" <- w382
            }
            frame "amplitude/offset" {
              n153 = Divide(x=w407, y=w406) -> (x/y=w405:dbl)
            }
          }
          n154 = Bundle By Name(cluster=w325, "best fit parameters"=w323) -> (w324:refnum<class "DAQOrcaFlash.lvclass">)
        }
        frame "5% brightest" {
          n155 = disable-structure shown="Disabled" {
            disable-tunnel: [w436 w437] -> w418
            disable-tunnel: w417 -> [w435 w437]
            disable-tunnel: w415 -> [w434 _]
            disable-tunnel: [w433 _] -> w414
            disable-tunnel: [w432 _] -> w413
            disable-tunnel: [w431 _] -> w412
            frame Disabled {
              # "Percentage of brightest pixel"
              # "Sorting takes about 600-700 ms for full frame (2048x2048)"
              n156 = Tick Count (ms)() -> (millisecond timer value=w420:u32)
              n157 = Array Size(array=dbl[] []) -> ()  [unwired: 1 out]
              n158 = To Double Precision Float(number=w420) -> (double precision float=w431:dbl)
              n159 = Multiply Array Elements() -> (0:w421:dbl)  [unwired: 1 in]
              n160 = Subtract(x=w431, y=w434) -> (x-y=w433:dbl)
              n161 = To Double Precision Float(number=w421) -> (double precision float=w427:dbl)
              n162 = Reshape Array(w421) -> ()  [unwired: 1 in, 1 out]
              n163 = Multiply(x=w427, y=0.005) -> (x*y=w425:dbl)
              n164 = Sort 1D Array() -> (sorted array=w428:dbl[])  [unwired: 1 in]
              n165 = To Long Integer(number=w425) -> (32bit integer=w424:i32)
              n166 = Subtract(x=w421, y=w424) -> (x-y=w423:dbl)
              n167 = Array Subset(array=w428, index=w423, length=w424) -> (w422:dbl[])
              n168 = To Double Precision Float(number=w422) -> (double precision float=w429:dbl[])
              n169 = call-poly <vilib>:"Mean.vi"("X"=w429) -> ("mean"=w432:dbl, "error"=w430:i32)
              n170 = call <vilib>:"Error Cluster From Error Code.vi"("error in (no error)"=w435, "error code (0)"=w430) -> ("error out"=w436:errorcluster)  [unwired: 7 in]
            }
            frame Enabled {
            }
          }
        }
      }
      "MF" <- w62
      "HP" <- w58
      "residue" <- w40
      "center" <- w42
      "offset" <- w44
      "amplitude" <- w43
      "standard deviation" <- w41
      "LP" <- w5
      "HP" <- w6
      "LP" <- w7
      n171 = call "Convert to Dynamic Data10"("Array"=w48) -> ("Dynamic Data Type"=w54:dynamicdata)  [unwired: 3 in]
      n172 = call "Convert to Dynamic Data9"("Array"=w47) -> ("Dynamic Data Type"=w53:dynamicdata)  [unwired: 3 in]
      n173 = call "Convert to Dynamic Data12"("Array"=w46) -> ("Dynamic Data Type"=w51:dynamicdata)  [unwired: 3 in]
      n174 = call "Convert to Dynamic Data11"("Array"=w45) -> ("Dynamic Data Type"=w50:dynamicdata)  [unwired: 3 in]
      n175 = call "Build XY Graph5"("Y Input"=w53, "X Input"=w54) -> ("XY Graph"=→"Raw data":cluster{"Y":dbl[], "Y":dbl[]}[])  [unwired: 3 in, 6 out]
      n176 = call "Build XY Graph6"("Y Input"=w50, "X Input"=w51) -> ("XY Graph"=→"Gauss":cluster{"Y":dbl[], "Y":dbl[]}[])  [unwired: 3 in, 6 out]
      n177 = Bundle By Name(cluster=w78, "MF abs time"=w77, "MF delta time"=w79, "Merit factor"=w62) -> (w64:refnum<class "DAQOrcaFlash.lvclass">)
      n178 = Format Into String(error in=w74, w62) -> (resulting string=w72:string, error out=w73:errorcluster)  [unwired: 2 in]
      n179 = call <vilib>:"Add or replace parameter.vi"("error in (no error)"=w73, "value"=w72, "name"="merit_factor", "Message in"=refnum<class "GenericMessage.lvclass"> refnum ("Distrio Murmex 1.5:GenericMessage")) -> ("error out"=w71:errorcluster, "Message out"=w70:refnum<class "GenericMessage.lvclass">)  [unwired: 6 in]
      n180 = call <vilib>:"Set generic command.vi"("error in (no error)"=w71, "generic command"="current_MF", "GenericMessage in"=w70) -> ("error out"=w75:errorcluster, "GenericMessage out"=w65:refnum<class "GenericMessage.lvclass">)  [unwired: 7 in]
      n181 = call <vilib>:"Send.vi"("error in (no error)"=w75, "Message"=w65, "recipient"="RSA" ("target ID"), "Murmex in"=w64) -> ("error out"=w67:errorcluster, "Murmex out"=w63:refnum<class "DAQOrcaFlash.lvclass">)  [unwired: 6 in]
    }
    frame Error {
    }
  }
  "error out" <- w4
  "DAQOrcaFlash out" <- w2
